vi "forwardByNavX_theSide(queuesWithNavX).vi"(5 "I2C Ref Out":T1, 8 "error in (no error)":errorcluster, 11 "distance the side":u32) -> (0 "error out":errorcluster, 2 "I2C Ref Out 2":T1)   [LabVIEW 2017]
uses:
  <vilib>/myRIO/Instrument Drivers/Onboard IO/I2C/typedefs/I2C Reference.ctl
  <vilib>/myRIO/Common/Instrument Driver Framework/Utilities/typedefs/myRIO Generic Hardware Reference.ctl
  <vilib>/myRIO/Common/Instrument Driver Framework/Utilities/typedefs/Hardware Version Enum.ctl
  <vilib>/myRIO/Common/Instrument Driver Framework/Utilities/typedefs/myRIO v1.0 Reference.ctl
  <vilib>/myRIO/Common/Instrument Driver Framework/Utilities/typedefs/Generic FPGA Reference.ctl
  <vilib>/myRIO/Common/Instrument Driver Framework/myRIO v1.0/I2C/typedefs/I2C Channels Enum.ctl
  <vilib>/myRIO/Instrument Drivers/Onboard IO/I2C/typedefs/I2C Configuration.ctl
  <vilib>/myRIO/Instrument Drivers/Onboard IO/I2C/typedefs/I2C Transfer Rate.ctl
  <vilib>/Instr/_visa.llb/VISA Configure Serial Port (Instr).vi
  <vilib>/Utility/error.llb/Error Cluster From Error Code.vi
  <vilib>/myRIO/Common/Instrument Driver Framework/myRIO v1.0/DIO/vis/myRIO v1.0 Write DIO.vi
  <vilib>/myRIO/Instrument Drivers/Onboard IO/DIO/DIO.lvlib
  <vilib>/myRIO/Instrument Drivers/Onboard IO/I2C/I2C.lvlib
panel:
  out "output 1":u32
  out "axis Z(paste)":ext
  out "main angle":ext
  out "right":dbl
  out "left":dbl
  out "zero angle":ext
  in  "Stop Button":bool
  out "axis Z(after)":ext
  # "--- отклонения от нулевого угла"
  # "PWM"
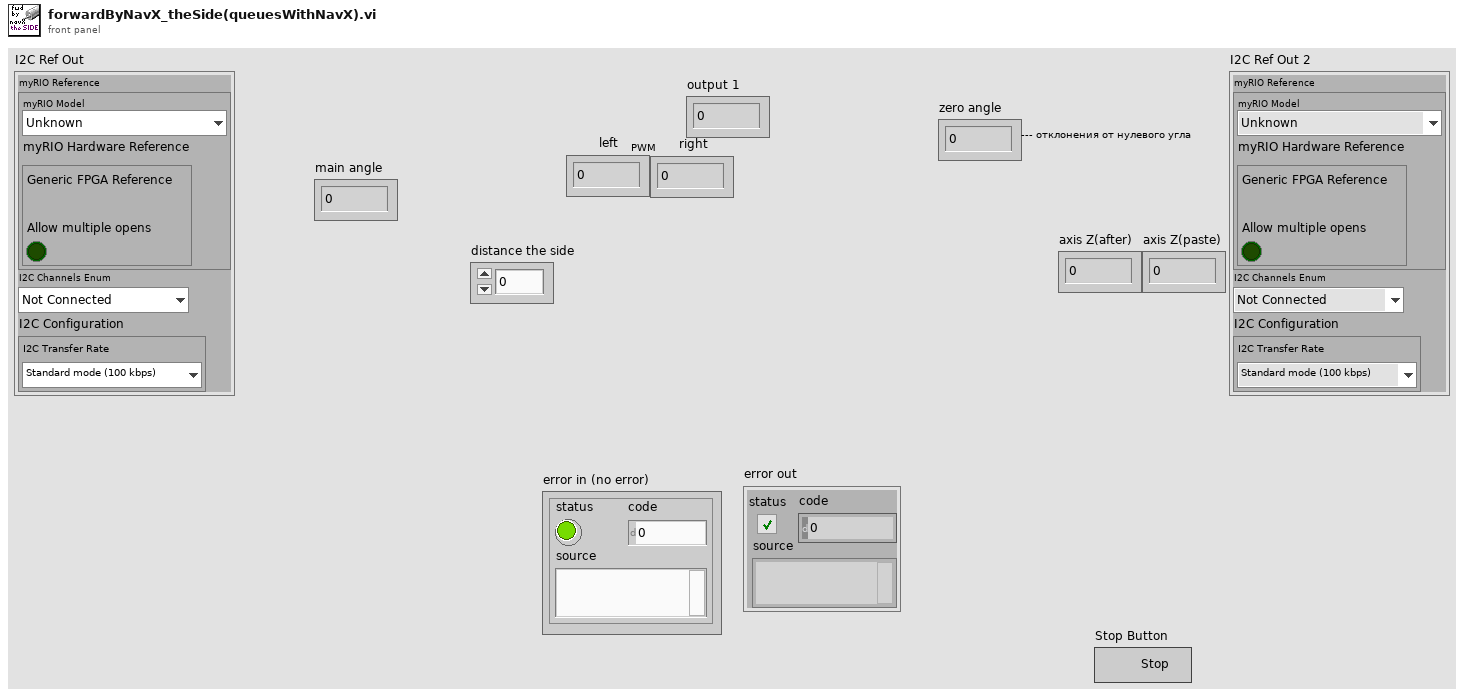
[diagram p1: front panel]
types:
  T1 = typedef "I2C.lvlib/I2C Reference.ctl" = cluster{"myRIO Reference":T2, "I2C Channels Enum":T6, "I2C Configuration":T7}
  T2 = typedef "myRIO Generic Hardware Reference.ctl" = cluster{"myRIO Model":T3, "myRIO Hardware Reference":T4}
  T3 = typedef "Hardware Version Enum.ctl" = enum16{"Unknown", "myRIO-1900", "myRIO-1950", "roboRIO", "NI ELVIS RIO CM"}
  T4 = typedef "myRIO v1.0 Reference.ctl" = cluster{"Generic FPGA Reference":T5, "Allow multiple opens":bool}
  T5 = typedef "Generic FPGA Reference.ctl" = refnum<k20>
  T6 = typedef "I2C Channels Enum.ctl" = enum16{"Not Connected", "A/I2C", "B/I2C", "I2C/I2C"}
  T7 = typedef "I2C.lvlib/I2C Configuration.ctl" = cluster{"I2C Transfer Rate":T8}
  T8 = typedef "I2C.lvlib/I2C Transfer Rate.ctl" = enum16{"Standard mode (100 kbps)", "Fast mode (400 kbps)"}
  T9 = typedef "DIO.lvlib/DIO Reference.ctl" = cluster{"myRIO Reference":T2, "DIO Channels List":T10}
  T10 = typedef "DIO Channels List.ctl" = T11[]
  T11 = typedef "DIO Channels Enum.ctl" = enum16{"Not Connected", "C/DIO0", "C/DIO1", "C/DIO2", "C/DIO3", "C/DIO4", "C/DIO5", "C/DIO6", "C/DIO7", "A/DIO0", "A/DIO1", "A/DIO2", "A/DIO3", "A/DIO4", "A/DIO5", "A/DIO6", "A/DIO7", "A/DIO8", "A/DIO9", "A/DIO10", "A/DIO11", "A/DIO12", "A/DIO13", "A/DIO14", "A/DIO15", "B/DIO0", "B/DIO1", "B/DIO2", "B/DIO3", "B/DIO4", "B/DIO5", "B/DIO6", "B/DIO7", "B/DIO8", "B/DIO9", "B/DIO10", "B/DIO11", "B/DIO12", "B/DIO13", "B/DIO14", "B/DIO15", "LED0", "LED1", "LED2", "LED3", "Button0", "DIO/DIO0", "DIO/DIO1", "DIO/DIO2", "DIO/DIO3", "DIO/DIO4", "DIO/DIO5", "DIO/DIO6", "DIO/DIO7", "DIO/DIO8", "DIO/DIO9", "SPI/CS0", "SPI/CS1", "SPI/CS2", "SPI/CS3", "LED RADIO (Green)", "LED RADIO (Red)", "LED COMM (Green)", "LED COMM (Red)", "LED MODE (Green)", "LED MODE (Red)"}
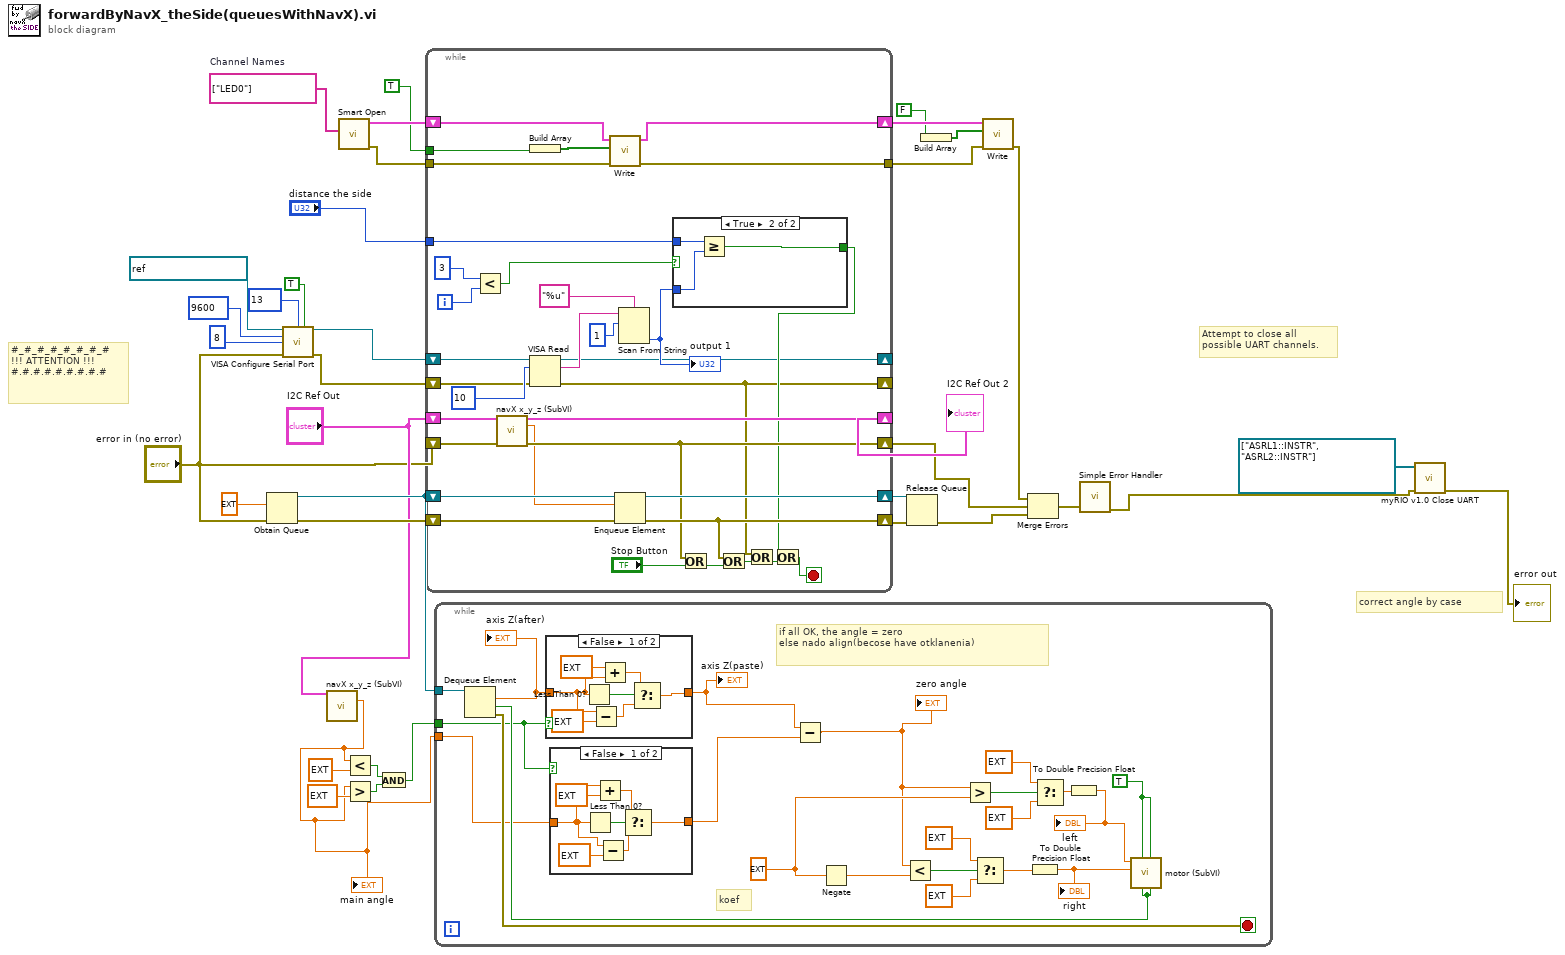
[diagram p0: block diagram]
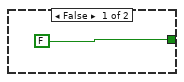
[diagram p4: hidden frame]
diagram:
  w12 = tag[] ["LED0"]  # Channel Names
  # "Attempt to close all possible UART channels."
  # "correct angle by case"
  # "#_#_#_#_#_#_#_#\n!!! ATTENTION !!!\n#.#.#.#.#.#.#.#.#"
  n1 = Obtain Queue(element data type=ext 0.0 ("value Z"), error in (no error)="error in (no error)") -> (queue out=w30:refnum<queue>, error out=w37:errorcluster)  [unwired: 3 in, 1 out]
  n2 = call-poly "VISA Configure Serial Port"("VISA resource name"=refnum<visa-resource-name> "ASRL2::INSTR" ("UART selector"), "termination char\n(0xA = '\\n' = LF)"=u8 13 ("termination char = CR"), "Enable Termination\nChar (T)"=TRUE ("enable termination char"), "baud rate (9600)"=u32 9600 ("baud rate"), "data bits (8)"=u16 8 ("data bits"), "error in (no error)"="error in (no error)") -> ("VISA resource name out"=w17:refnum<visa-resource-name>, "error out"=w18:errorcluster)  [unwired: 8 in]
  n3 = call "navX x_y_z (SubVI).vi"("I2C Ref Out in"="I2C Ref Out") -> ("value Z"=w27:ext)  [unwired: 10 in, 4 out]
  "main angle" <- w27
  n4 = call <vilib>:"Smart Open.vi"("Channel Names"=w12) -> ("error out"=w10:errorcluster, "DIO Ref Out"=w11:T9)  [unwired: 9 in]
  n5 = Less?(x=w27, y=ext 90.0) -> (x < y?=w25:bool)
  n6 = Greater?(x=w27, y=ext -90.0) -> (0:w28:bool)
  n7 = And(x=w25, y=w28) -> (x .and. y?=w24:bool)
  n8 = while {
    shift-right: [w65] -> w35
    shift-left: w37 -> [w70]
    shift-right: [w69] -> w36
    shift-left: w30 -> [w71]
    shift-right: [w66] -> w33
    shift-left: "I2C Ref Out" -> [w67]
    shift-right: [w62] -> w1
    shift-left: "error in (no error)" -> [w63]
    tunnel: "distance the side" -> [w49]
    shift-right: [w45] -> _
    shift-left: w18 -> [w51]
    shift-right: [w47] -> _
    shift-left: w17 -> [w50]
    tunnel: w10 -> [w41]
    tunnel: TRUE -> [w40]
    tunnel: [w38] -> w5
    shift-right: [w39] -> w8
    shift-left: w11 -> [w42]
    i -> [w44]
    stop <- w59 stop-if-true
    n9 = Less?(x=3, y=w44) -> (x < y?=w52:bool)
    n10 = call "navX x_y_z (SubVI).vi"("I2C Ref Out in"=w67, "error in (no error)"=w63) -> ("I2C Ref Out out"=w66:T1, "value Z"=w61:ext, "error out"=w62:errorcluster)  [unwired: 9 in, 2 out]
    n11 = Build Array(w40) -> (w43:bool[])
    n12 = VISA Read(VISA resource name=w50, byte count=u32 10, error in (no error)=w51) -> (VISA resource name out=w47:refnum<visa-resource-name>, read buffer=w55:string, error out=w45:errorcluster)  [unwired: 1 out]
    n13 = call <vilib>:"Write.vi"("error in (no error)"=w41, "Values"=w43, "DIO Ref In"=w42) -> ("error out"=w38:errorcluster, "DIO Ref Out"=w39:T9)  [unwired: 6 in]
    n14 = Enqueue Element(queue=w71, element=w61, error in (no error)=w70) -> (queue out=w69:refnum<queue>, error out=w65:errorcluster)  [unwired: 1 in, 1 out]
    n15 = Scan From String(format string="%u", input string=w55, initial scan location=u32 1) -> (output 1=w54:u32)  [unwired: 2 in, 3 out]
    "output 1" <- w54
    n16 = case shown="True" w52 {
      tunnel: w54 -> [_ w75]
      tunnel: w49 -> [_ w74]
      tunnel: [FALSE w73] -> w48
      frame False {
      }
      frame True {
        n17 = Greater Or Equal?(x=w74, y=w75) -> (x >= y?=w73:bool)
      }
    }
    n18 = Or(x=w62, y="Stop Button") -> (x .or. y?=w64:bool)
    n19 = Or(x=w65, y=w64) -> (x .or. y?=w60:bool)
    n20 = Or(x=w45, y=w60) -> (x .or. y?=w46:bool)
    n21 = Or(x=w48, y=w46) -> (x .or. y?=w59:bool)
  }
  "I2C Ref Out 2" <- w33
  n22 = while {
    tunnel: w30 -> [w97]
    tunnel: w27 -> [w79]
    tunnel: w24 -> [w78]
    stop <- w96 stop-if-true
    w85 = TRUE ("M0 (Pin 21)")
    w89 = ext 1.0 ("y")
    # "koef"
    # "if all OK, the angle = zero\nelse nado align(becose have otklanenia)"
    n23 = Dequeue Element(queue=w97) -> (element=w81:ext, timed out?=w84:bool, error out=w96:errorcluster)  [unwired: 2 in, 1 out]
    "axis Z(after)" <- w81
    n24 = case shown="False" w78 {
      tunnel: [w111 w113] -> w82
      tunnel: w81 -> [w107 w113]
      frame False {
        n25 = Less Than 0?(x=w107) -> (x < 0?=w112:bool)
        n26 = Subtract(x=w107, y=ext 180.0) -> (x-y=w108:ext)
        n27 = Add(x=ext 180.0, y=w107) -> (x+y=w110:ext)
        n28 = Select(t=w110, s=w112, f=w108) -> (s? t:f=w111:ext)
      }
      frame True {
      }
    }
    "axis Z(paste)" <- w82
    n29 = case shown="False" w78 {
      tunnel: [w103 w105] -> w80
      tunnel: w79 -> [w100 w105]
      frame False {
        n30 = Less Than 0?(x=w100) -> (x < 0?=w104:bool)
        n31 = Add(x=w100, y=ext 180.0) -> (x+y=w102:ext)
        n32 = Subtract(x=w100, y=ext 180.0) -> (x-y=w101:ext)
        n33 = Select(t=w102, s=w104, f=w101) -> (s? t:f=w103:ext)
      }
      frame True {
      }
    }
    n34 = Subtract(x=w82, y=w80) -> (x-y=w83:ext)
    "zero angle" <- w83
    n35 = Negate(x=w89) -> (-x=w88:ext)
    n36 = Less?(x=w83, y=w88) -> (x < y?=w92:bool)
    n37 = Greater?(x=w83, y=w89) -> (0:w95:bool)
    n38 = Select(t=ext 0.2 ("y"), s=w92, f=ext 0.4 ("y")) -> (s? t:f=w86:ext)
    n39 = To Double Precision Float(number=w86) -> (double precision float=w77:dbl)
    "right" <- w77
    n40 = Select(t=ext 0.2 ("y"), s=w95, f=ext 0.4 ("y")) -> (s? t:f=w87:ext)
    n41 = To Double Precision Float(number=w87) -> (double precision float=w76:dbl)
    "left" <- w76
    n42 = call "motor (SubVI).vi"("M1 (Pin 26)"=w84, "M1 (Pin 25)"=w85, "M0 (Pin 23)"=w84, "M0 (Pin 21)"=w85, "PWM1"=w77, "PWM0"=w76) -> ()  [unwired: 5 in, 1 out]
  }
  n43 = Release Queue(queue=w36, error in (no error)=w35) -> (error out=w31:errorcluster)  [unwired: 1 in, 2 out]
  n44 = Build Array(FALSE) -> (w7:bool[])
  n45 = call <vilib>:"Write.vi"("error in (no error)"=w5, "Values"=w7, "DIO Ref In"=w8) -> ("error out"=w4:errorcluster)  [unwired: 6 in, 1 out]
  n46 = Merge Errors(w4, w1, w31) -> (w32:errorcluster)
  n47 = call <vilib>:"Simple Error Handler.vi"("error in (no error)"=w32) -> ("error out"=w14:errorcluster)  [unwired: 4 in, 4 out]
  n48 = call <vilib>:"myRIO v1.0 Close UART.vi"("error in (no error)"=w14, "VISA resource array"=refnum<visa-resource-name>[] ["ASRL1::INSTR", "ASRL2::INSTR"]) -> ("error out"=→"error out":errorcluster)  [unwired: 9 in]
